vi "Read DO Lines.vi"(8 "error in (no error)":errorcluster, 11 "Set Output Lines Msg in":refnum<class "Set Output Lines Msg.lvclass">) -> (0 "error out":errorcluster, 2 "DO Lines":bool[](array[boolean]), 3 "Set Output Lines Msg out":refnum<class "Set Output Lines Msg.lvclass">)   [LabVIEW 2016, in "BNT_DAQmx.lvlib" / "Set Output Lines Msg.lvclass"]
uses:
  Set Output Lines Msg.lvclass
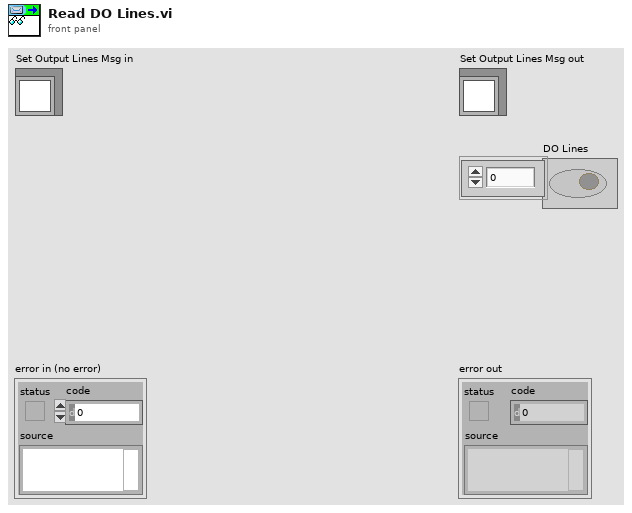
[diagram p1: front panel]
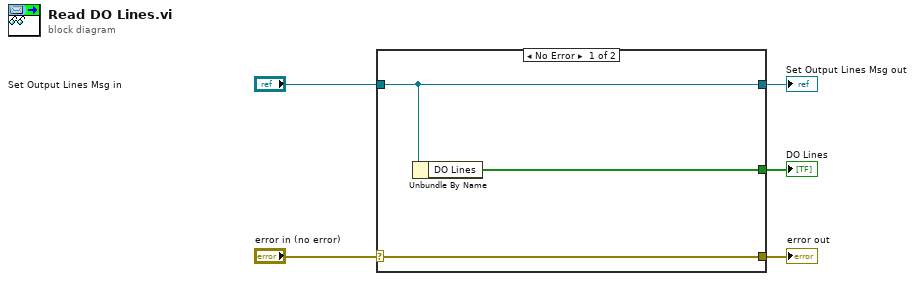
[diagram p0: block diagram]
diagram:
  n1 = case shown="No Error" "error in (no error)" {
    selector: "error in (no error)" -> [w8 w9]
    tunnel: [w8 w9] -> w4
    tunnel: [w7 w10] -> w2
    tunnel: "Set Output Lines Msg in" -> [w7 w10]
    tunnel: [w6 _] -> w1
    frame No Error {
      n2 = Unbundle By Name(w7) -> ("DO Lines"=w6:bool[])
    }
    frame Error {
    }
  }
  "error out" <- w4
  "Set Output Lines Msg out" <- w2
  "DO Lines" <- w1
